vi "Test - Read Waveform.vi"() -> ()   [LabVIEW 2020]
uses:
  RTL-SDR/Device/Device.lvclass
  RTL-SDR/Session/Session.lvclass
  RTL-SDR/Session/Read Samples (Complex DBL Waveform).vi
panel:
  out "Graph":cluster{"x0":dbl, "dx":dbl, "[y]":dbl[]}(graph)
  in  "Sample Rate":u32=1000000 step=10000 format="%#.12p"
  in  "Center Frequency":u32=434000000 step=10000 format="%#.12p"
  out "Serial":string
  out "Product":string
  out "Mfg":string
  out "Name":string
  out "s":dbl
  in  "stop":bool
  out "Actual Sample Rate":u32 format="%#.12f"
  out "Actual Center Frequency":u32 format="%#.12p"
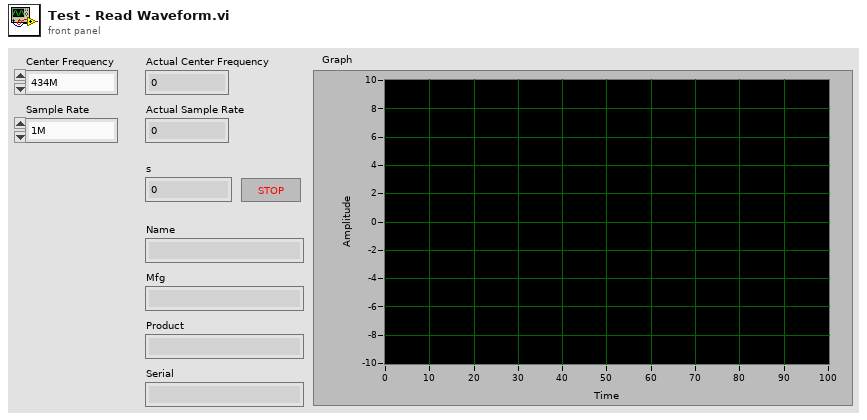
[diagram p1: front panel]
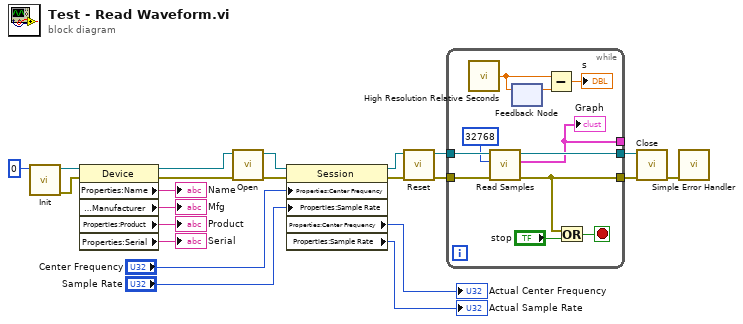
[diagram p0: block diagram]
diagram:
  n1 = call "Init.vi"("Index"=0) -> ("error out"=w20:errorcluster, "Device out"=w21:refnum<class "Device.lvclass">)  [unwired: 9 in]
  n2 = property class="Device"(reference=w21, error in=w20) -> (reference out=w18:refnum<class "Device.lvclass">, error out=w19:errorcluster, "Properties:Name"=→"Name":string, "Properties:Manufacturer"=→"Mfg":string, "Properties:Product"=→"Product":string, "Properties:Serial"=→"Serial":string)
  n3 = call "Open.vi"("error in (no error)"=w19, "Device"=w18) -> ("error out"=w14:errorcluster, "RTL-SDR out"=w3:refnum<class "Session.lvclass">)  [unwired: 8 in]
  n4 = property class="Session"(reference=w3, error in=w14, "Properties:Center Frequency"="Center Frequency", "Properties:Sample Rate"="Sample Rate") -> (reference out=w10:refnum<class "Session.lvclass">, error out=w11:errorcluster, "Properties:Center Frequency"=→"Actual Center Frequency":u32, "Properties:Sample Rate"=→"Actual Sample Rate":u32)
  n5 = call "Reset.vi"("error in (no error)"=w11, "RTL-SDR in"=w10) -> ("error out"=w8:errorcluster, "RTL-SDR out"=w9:refnum<class "Session.lvclass">)  [unwired: 8 in]
  n6 = while {
    tunnel: w9 -> [w28]
    tunnel: w8 -> [w27]
    tunnel: [w25] -> w17
    tunnel: [w26] -> w16
    tunnel: [w23] -> _
    stop <- w32 stop-if-true
    n7 = call <vilib>:"High Resolution Relative Seconds.vi"() -> ("relative seconds"=w30:dbl)
    n8 = call-poly "Read Samples.vi"("error in (no error)"=w27, "Samples"=32768, "RTL-SDR in"=w28) -> ("error out"=w26:errorcluster, "Complex DBL Waveform"=w23:cluster{"x0":dbl, "dx":dbl, "[y]":cdb[]}, "RTL-SDR out"=w25:refnum<class "Session.lvclass">)  [unwired: 6 in]
    "Graph" <- w23
    n9 = feedback-in #1(w30) -> ()
    n10 = feedback #1() -> (w31:dbl)  [unwired: 1 in]
    n11 = Subtract(x=w30, y=w31) -> (x-y=→"s":dbl)
    n12 = Or(x=w26, y="stop") -> (x .or. y?=w32:bool)
  }
  n13 = call "Close.vi"("error in (no error)"=w16, "RTL-SDR in"=w17) -> ("error out"=w15:errorcluster)  [unwired: 8 in, 1 out]
  n14 = call <vilib>:"Simple Error Handler.vi"("error in (no error)"=w15) -> ()  [unwired: 4 in, 5 out]
